vi "Configure.vi"(8 "error in (no error)":errorcluster, 11 "DAQMH121119OrcaFlash in":refnum<class "DAQOrcaFlash.lvclass">) -> (0 "error out":errorcluster, 2 "cancelled?":bool, 3 "DAQMH121119OrcaFlash out":refnum<class "DAQOrcaFlash.lvclass">)   [LabVIEW 2012, in "DAQOrcaFlash.lvclass"]
doc: "The configure method configures the details for the RabbitMQ connection. \n\nIn the derived class, make a call to the parent for setting these parameters."
uses:
  DAQOrcaFlash.lvclass
  trigger_source.ctl
  read out direction.ctl
  sensor_mode.ctl
  trigger_mode.ctl
  output trigger type.ctl
  connector.ctl
  output trigger period.ctl
  trigger_polarity.ctl
  <vilib>/Utility/miscctls.llb/LVPointTypeDef.ctl
  DAQOrcaFlash.lvclass/DAQOrcaFlash.ctl
  <vilib>/Distrio/Murmex/Murmex/Murmex.lvclass
  output trigger source.ctl
panel:
  in  "Tab Control":T1(tab)=enum."Trigger"
  in  "Sensor mode":T2=12.0 items=["Normal"=1, "Light sheet"=12]
  in  "Read out direction":T3=1.0 items=["Top to Bottom"=1, "Bottom to Top"=2]
  in  "Trigger polarity":T4 items=["Negative"=1, "Positive"=2]
  in  "Output trigger period":T5=1e-05 min=5e-06 max=10 format="%#_6e"
  in  "Output trigger connector":T6=enum."3"
  in  "Output trigger type":T7=1.0 items=["Low"=1, "Global exposure"=2, "Programmable"=3, "Trigger ready"=4, "High"=5]
  in  "Trigger mode":T8=1.0 items=["Normal"=1, "Start"=6]
  in  "Trigger source":T9=2.0 items=["Internal"=1, "External"=2, "Software"=3]
  in  "Output trigger source":sgl(ring)=2.0 items=["READOUTEND"=2, "VSYNC"=3, "HSYNC"=4]
  in  "Output trigger polarity":T4 items=["Negative"=1, "Positive"=2]
  in  "relay start/stop to...":i32(listbox)
  in  "button:removeRelayTarget":bool
  in  "button:addRelayTarget":bool
  in  "relay target ID":string caption="target component ID"
  in  "conversion directory":path=path "R:/test_hamamatsu"
  in  "storage directory":path=path "R:/test_hamamatsu"
  in  "enable start buttons?":bool
  in  "maximum window size":dbl=1024.0 caption="px"
  in  "Autofocus component":string
  in  "Tomo component":string
  in  "Stack component":string
  in  "button:cancel":bool
  in  "button:ok":bool
  in  "button:configure_murmex":bool
  # "input Trigger"
  # "output trigger"
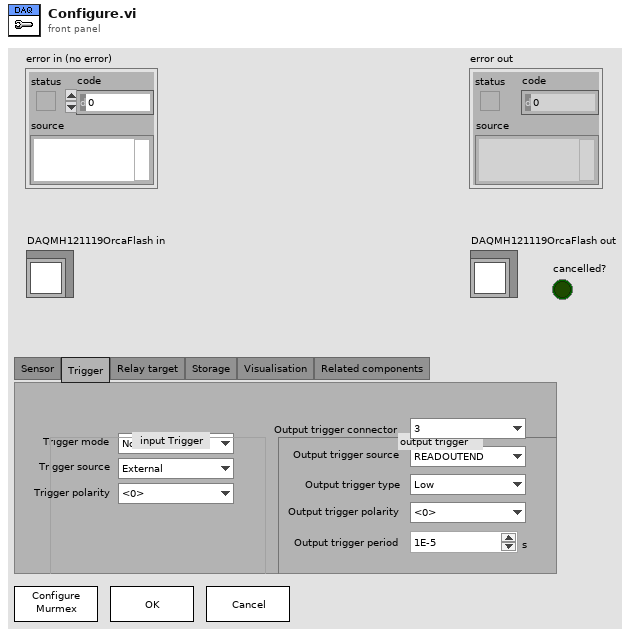
[diagram p1: front panel]
types:
  T1 = enum32{"Sensor", "Trigger", "Relay target", "Storage", "Visualisation", "Related components"}
  T2 = typedef "DAQOrcaFlash.lvclass/sensor_mode.ctl" = sgl
  T3 = typedef "DAQOrcaFlash.lvclass/read out direction.ctl" = sgl
  T4 = typedef "DAQOrcaFlash.lvclass/trigger_polarity.ctl" = sgl
  T5 = typedef "DAQOrcaFlash.lvclass/output trigger period.ctl" = sgl[unit]
  T6 = typedef "DAQOrcaFlash.lvclass/connector.ctl" = enum32{"1", "2", "3"}
  T7 = typedef "DAQOrcaFlash.lvclass/output trigger type.ctl" = sgl
  T8 = typedef "DAQOrcaFlash.lvclass/trigger_mode.ctl" = sgl
  T9 = typedef "DAQOrcaFlash.lvclass/trigger_source.ctl" = sgl
  T10 = enum32{"Sensor", "Trigger", "Relay target", "Storage"}
  T11 = typedef "LVPointTypeDef.ctl" = cluster{"Horizontal":i16, "Vertical":i16}
  T12 = typedef "DAQOrcaFlash.lvclass/output trigger source.ctl" = sgl
  T13 = enum8{"Enabled", "Disabled", "Disabled and Grayed Out"}
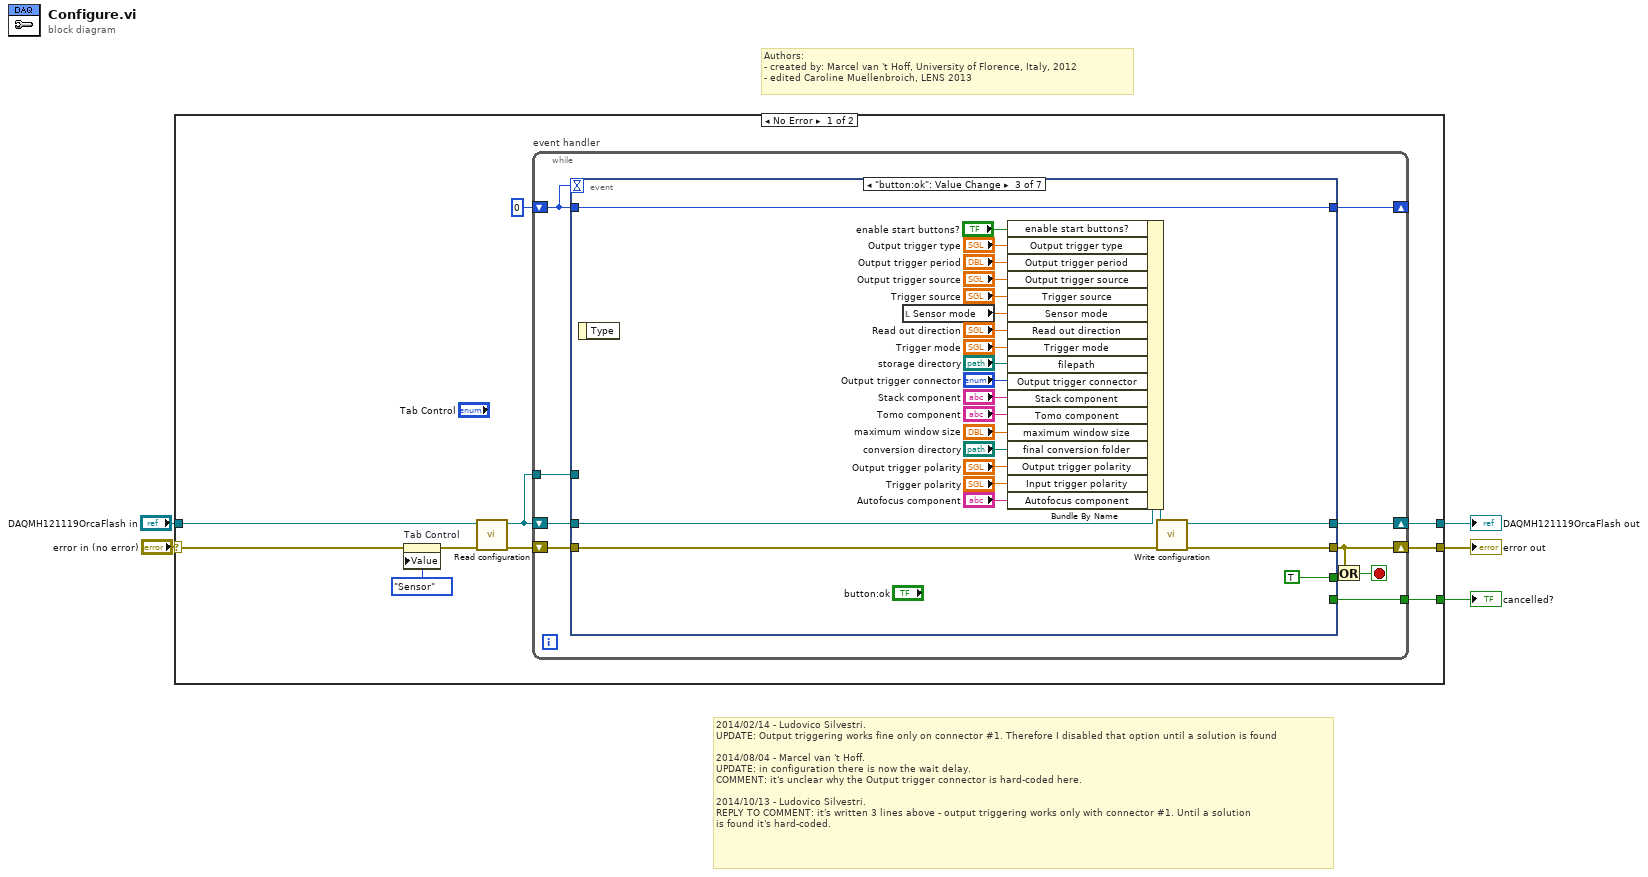
[diagram p0: block diagram]
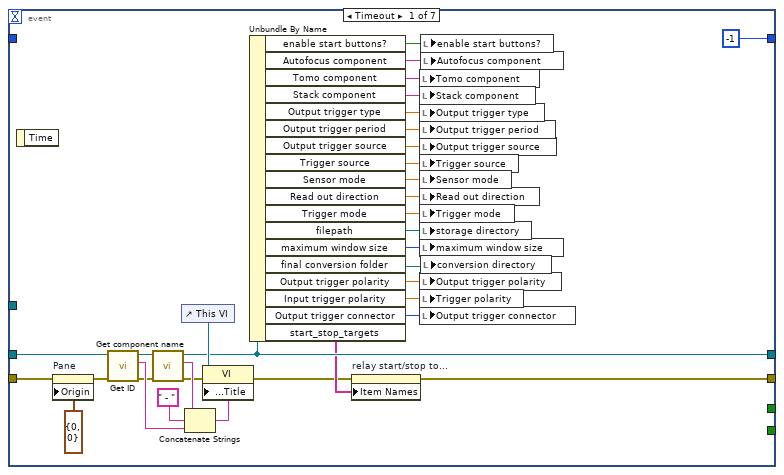
[diagram p2: hidden frame]
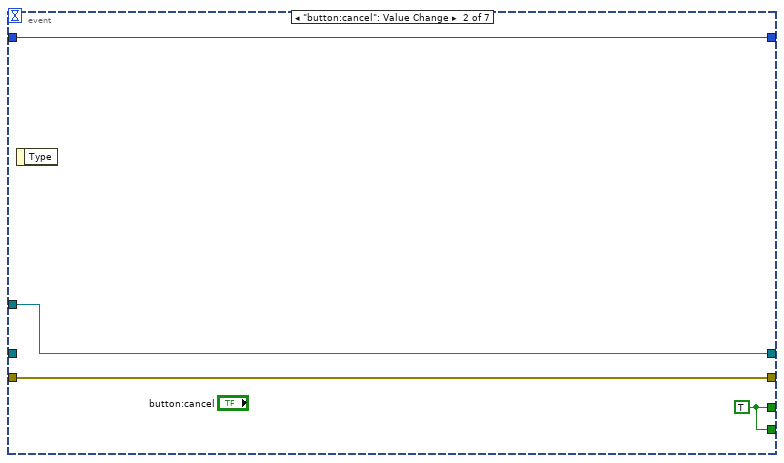
[diagram p3: hidden frame]
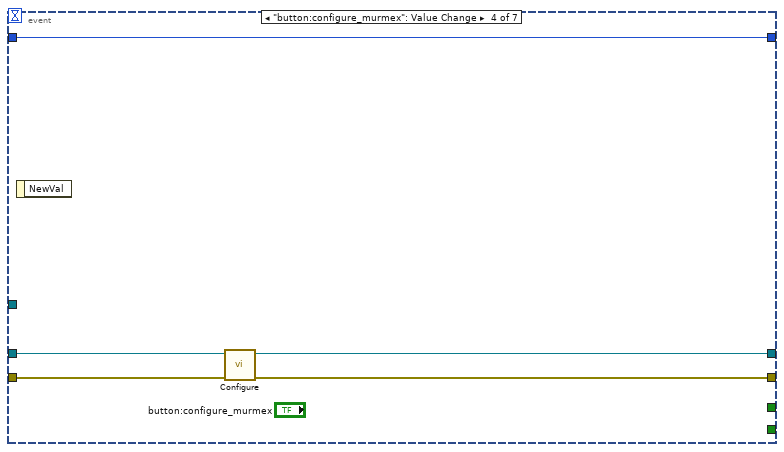
[diagram p4: hidden frame]
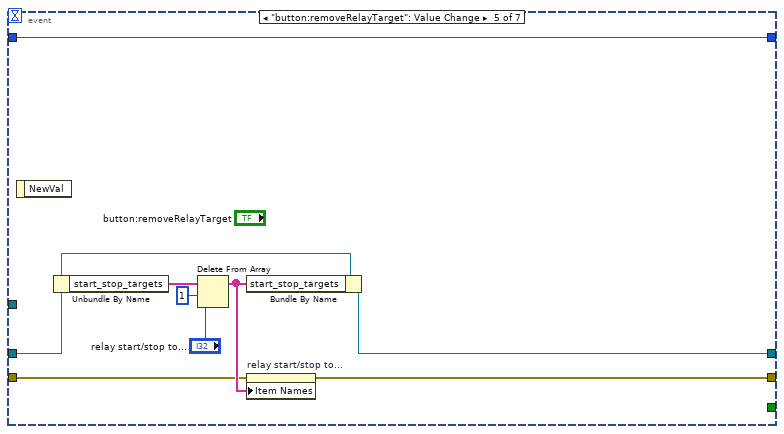
[diagram p5: hidden frame]
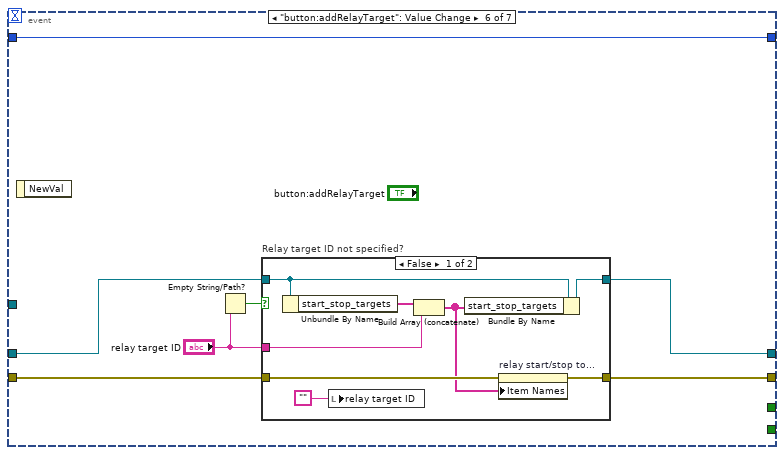
[diagram p6: hidden frame]
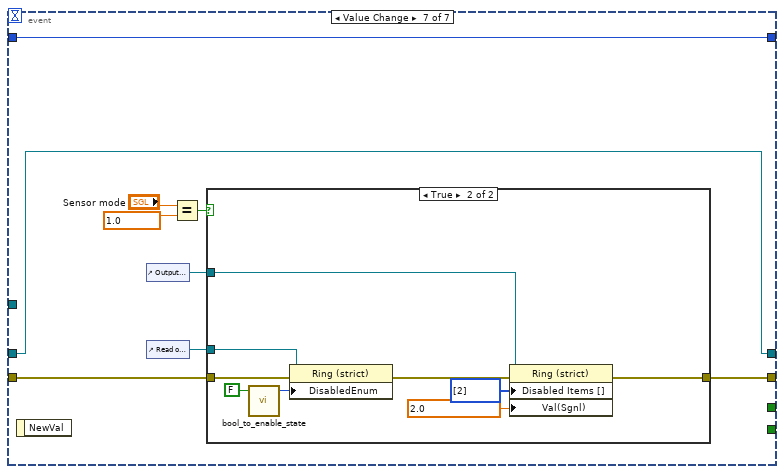
[diagram p8: hidden frame]
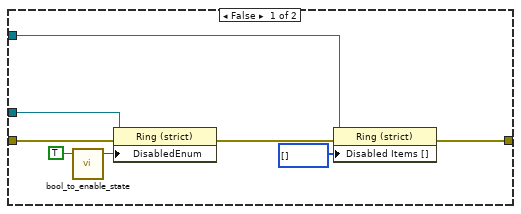
[diagram p9: hidden frame]
diagram:
  # "2014/02/14 - Ludovico Silvestri.\nUPDATE: Output triggering works fine only on connector #1. Therefore I disabled that option until a solution is found\n\n2014/08/04 - Marcel van 't Hoff.\nUPDATE: in configuration there is now the wait delay.\nCOMMENT: it's unclear why the Output trigger connector is hard-coded here.\n\n2014/10/13 - Ludovico Silvestri.\nREPLY TO COMMENT: it's written 3 lines above - output triggering works only with connector #1. Until a solution\nis found it's hard-coded."
  # "Authors: \n- created by: Marcel van 't Hoff, University of Florence, Italy, 2012\n- edited Caroline Muellenbroich, LENS 2013"
  n1 = case shown="No Error" "error in (no error)" {
    selector: "error in (no error)" -> [w7 w145]
    tunnel: [w15 w145] -> w5
    tunnel: [w14 w146] -> w1
    tunnel: [w12 _] -> w4
    tunnel: "DAQMH121119OrcaFlash in" -> [w10 w146]
    frame No Error {
      n2 = property on="Tab Control" class="TabCtl (strict)"(error in=w7, "Value"=T10."Sensor" ("Tab Control")) -> (error out=w6:errorcluster)  [unwired: 1 in, 1 out]
      n3 = call <vilib>:"Read configuration.vi"("error in (no error)"=w6, "Murmex in"=w10) -> ("error out"=w11:errorcluster, "Murmex out"=w9:refnum<class "DAQOrcaFlash.lvclass">)  [unwired: 7 in, 1 out]
      n4 = while "event handler" {
        shift-right: [w22] -> w15
        shift-left: w11 -> [w24]
        shift-right: [w25] -> w14
        shift-left: w9 -> [w23]
        shift-right: [w20] -> _
        shift-left: 0 -> [w19]
        tunnel: [w17] -> w12
        tunnel: w9 -> [w16]
        stop <- w21 stop-if-true
        n5 = event shown="[2] \"button:ok\": Value Change" {
          selector: _ -> [_ _ _ _ _ _ _]
          dyn-events: _ -> [_ _ _ _ _ _ _]
          timeout: w19 -> [_ _ _ _ _ _ _]
          tunnel: [w35 w63 w84 w92 w94 w103 w120] -> w22
          tunnel: [w38 w60 w83 w91 w98 w105 w119] -> w25
          tunnel: w24 -> [w56 w63 w87 w90 w95 w104 w123]
          tunnel: w23 -> [w59 _ w82 w89 w99 w106 w119]
          tunnel: [-1 w62 w86 w88 w93 w102 w127] -> w20
          tunnel: w19 -> [_ w62 w86 w88 w93 w102 w127]
          tunnel: [_ w61 TRUE _ _ _ _] -> w18
          tunnel: [_ w61 _ _ _ _ _] -> w17
          tunnel: w16 -> [_ w60 _ _ _ _ _]
          event Timeout {
            n6 = event-data() -> ()  [unwired: 1 in, 1 out]
            n7 = property on="Pane" class="Pane"(error in=w56, "Origin"=T11 {"Horizontal"=0, "Vertical"=0}) -> (error out=w51:errorcluster)  [unwired: 1 in, 1 out]
            n8 = call <vilib>:"Get ID.vi"("error in (no error)"=w51, "Murmex in"=w59) -> ("error out"=w50:errorcluster, "component id"=w53:string, "Murmex out"=w55:refnum<class "DAQOrcaFlash.lvclass">)  [unwired: 7 in]
            n9 = call <vilib>:"Get component name.vi"("error in (no error)"=w50, "Murmex in"=w55) -> ("error out"=w39:errorcluster, "component name"=w54:string, "Murmex out"=w38:refnum<class "DAQOrcaFlash.lvclass">)  [unwired: 7 in]
            n10 = control-ref of="This VI"() -> (w40:refnum<vi>)
            n11 = Concatenate Strings(w54, " - " ("string"), w53) -> (w41:string)
            n12 = property class="VI"(reference=w40, error in=w39, "Front Panel.Title"=w41) -> (error out=w36:errorcluster)  [unwired: 1 out]
            n13 = Unbundle By Name(w38) -> ("enable start buttons?"=w26:bool, "Autofocus component"=w28:string, "Tomo component"=w33:string, "Stack component"=w34:string, "Output trigger type"=w42:T7, "Output trigger period"=w43:sgl[unit], "Output trigger source"=w44:T12, "Trigger source"=w48:T9, "Sensor mode"=w47:T2, "Read out direction"=w46:T3, "Trigger mode"=w45:T8, "filepath"=w49:path, "maximum window size"=w32:i32, "final conversion folder"=w31:path, "Output trigger polarity"=w30:T4, "Input trigger polarity"=w29:T4, "Output trigger connector"=w27:T6, "start_stop_targets"=w37:string[])
            n14 = property on="relay start/stop to..." class="LstBox (strict)"(error in=w36, "Item Names"=w37) -> (error out=w35:errorcluster)  [unwired: 1 in, 1 out]
            n15 = local write "Tomo component"(w33) -> ()
            n16 = local write "Stack component"(w34) -> ()
            n17 = local write "Output trigger type"(w42) -> ()
            n18 = local write "Output trigger period"(w43) -> ()
            n19 = local write "Output trigger source"(w44) -> ()
            n20 = local write "Trigger source"(w48) -> ()
            n21 = local write "Sensor mode"(w47) -> ()
            n22 = local write "Read out direction"(w46) -> ()
            n23 = local write "Trigger mode"(w45) -> ()
            n24 = local write "storage directory"(w49) -> ()
            n25 = local write "maximum window size"(w32) -> ()
            n26 = local write "Output trigger polarity"(w30) -> ()
            n27 = local write "Trigger polarity"(w29) -> ()
            n28 = local write "Output trigger connector"(w27) -> ()
            n29 = local write "enable start buttons?"(w26) -> ()
            n30 = local write "Autofocus component"(w28) -> ()
            n31 = local write "conversion directory"(w31) -> ()
          }
          event "button:cancel": Value Change {
            w61 = TRUE
            n32 = event-data() -> ()  [unwired: 1 in, 1 out]
          }
          event "button:ok": Value Change {
            n33 = event-data() -> ()  [unwired: 1 in, 1 out]
            n34 = local read "Sensor mode"() -> (w73:T2)
            n35 = Bundle By Name(cluster=w82, "enable start buttons?"="enable start buttons?", "Output trigger type"="Output trigger type", "Output trigger period"="Output trigger period", "Output trigger source"="Output trigger source", "Trigger source"="Trigger source", "Sensor mode"=w73, "Read out direction"="Read out direction", "Trigger mode"="Trigger mode", "filepath"="storage directory", "Output trigger connector"="Output trigger connector", "Stack component"="Stack component", "Tomo component"="Tomo component", "maximum window size"="maximum window size", "final conversion folder"="conversion directory", "Output trigger polarity"="Output trigger polarity", "Input trigger polarity"="Trigger polarity", "Autofocus component"="Autofocus component") -> (w81:refnum<class "DAQOrcaFlash.lvclass">)
            n36 = call <vilib>:"Write configuration.vi"("error in (no error)"=w87, "Murmex in"=w81) -> ("error out"=w84:errorcluster, "Murmex out"=w83:refnum<class "DAQOrcaFlash.lvclass">)  [unwired: 8 in]
          }
          event "button:configure_murmex": Value Change {
            n37 = event-data() -> ()  [unwired: 1 in, 1 out]
            n38 = call-parent "Configure.vi"("error in (no error)"=w90, "Murmex in"=w89) -> ("error out"=w92:errorcluster, "Murmex out"=w91:refnum<class "DAQOrcaFlash.lvclass">)  [unwired: 7 in, 1 out]
          }
          event "button:removeRelayTarget": Value Change {
            n39 = event-data() -> ()  [unwired: 1 in, 1 out]
            n40 = Unbundle By Name(w99) -> ("start_stop_targets"=w101:string[])
            n41 = Delete From Array(array=w101, length=1, index="relay start/stop to...") -> (array with subset deleted=w96:string[])  [unwired: 1 out]
            n42 = Bundle By Name(cluster=w99, "start_stop_targets"=w96) -> (w98:refnum<class "DAQOrcaFlash.lvclass">)
            n43 = property on="relay start/stop to..." class="LstBox (strict)"(error in=w95, "Item Names"=w96) -> (error out=w94:errorcluster)  [unwired: 1 in, 1 out]
          }
          event "button:addRelayTarget": Value Change {
            n44 = event-data() -> ()  [unwired: 1 in, 1 out]
            n45 = Empty String/Path?(string/path="relay target ID") -> (empty?=w108:bool)
            n46 = case "Relay target ID not specified?" shown="False" w108 {
              tunnel: w106 -> [w115 w118]
              tunnel: [w114 w118] -> w105
              tunnel: "relay target ID" -> [w113 _]
              tunnel: w104 -> [w111 w117]
              tunnel: [w110 w117] -> w103
              frame False {
                n47 = Unbundle By Name(w115) -> ("start_stop_targets"=w116:string[])
                n48 = local write "relay target ID"("") -> ()
                n49 = Build Array (concatenate)(w116, w113) -> (w109:string[])
                n50 = Bundle By Name(cluster=w115, "start_stop_targets"=w109) -> (w114:refnum<class "DAQOrcaFlash.lvclass">)
                n51 = property on="relay start/stop to..." class="LstBox (strict)"(error in=w111, "Item Names"=w109) -> (error out=w110:errorcluster)  [unwired: 1 in, 1 out]
              }
              frame True {
              }
            }
          }
          event Value Change {
            w125 = T2 1.0 items=["Normal"=1.0, "Light sheet"=12.0] ("y")
            n52 = event-data() -> ()  [unwired: 1 in, 1 out]
            n53 = control-ref of="Output trigger source"() -> (w121:refnum<vi>)
            n54 = control-ref of="Read out direction"() -> (w122:refnum<vi>)
            n55 = Equal?(x="Sensor mode", y=w125) -> (x = y?=w124:bool)
            n56 = case shown="True" w124 {
              tunnel: w123 -> [w132 w143]
              tunnel: w122 -> [w131 w144]
              tunnel: w121 -> [w130 w140]
              tunnel: [w128 w138] -> w120
              frame False {
                n57 = call "bool_to_enable_state.vi"("boolean in"=TRUE) -> ("enabled status out"=w135:T13)  [unwired: 4 in]
                n58 = property class="Ring (strict)"(reference=w131, error in=w132, "DisabledEnum"=w135) -> (error out=w133:errorcluster)  [unwired: 1 out]
                n59 = property class="Ring (strict)"(reference=w130, error in=w133, "Disabled Items []"=i32[] []) -> (error out=w128:errorcluster)  [unwired: 1 out]
              }
              frame True {
                w136 = T12 2.0 items=["READOUTEND"=2.0, "VSYNC"=3.0, "HSYNC"=4.0] ("Value (Signaling)")
                n60 = call "bool_to_enable_state.vi"("boolean in"=FALSE) -> ("enabled status out"=w142:T13)  [unwired: 4 in]
                n61 = property class="Ring (strict)"(reference=w144, error in=w143, "DisabledEnum"=w142) -> (error out=w139:errorcluster)  [unwired: 1 out]
                n62 = property class="Ring (strict)"(reference=w140, error in=w139, "Disabled Items []"=i32[] [2], "Val(Sgnl)"=w136) -> (error out=w138:errorcluster)  [unwired: 1 out]
              }
            }
          }
        }
        n63 = Or(x=w22, y=w18) -> (x .or. y?=w21:bool)
      }
    }
    frame Error {
    }
  }
  "error out" <- w5
  "DAQMH121119OrcaFlash out" <- w1
  "cancelled?" <- w4
